vi "WriteUCharImageAttribute.vi"(2 "value":u8[][](array[numeric]), 3 "attribute name":string, 4 "device name":string) -> (0 "error stack":string[](array[string]), 1 "success":bool)   [LabVIEW 2014, in "tango.lvlib"]
uses:
  tango.lvlib
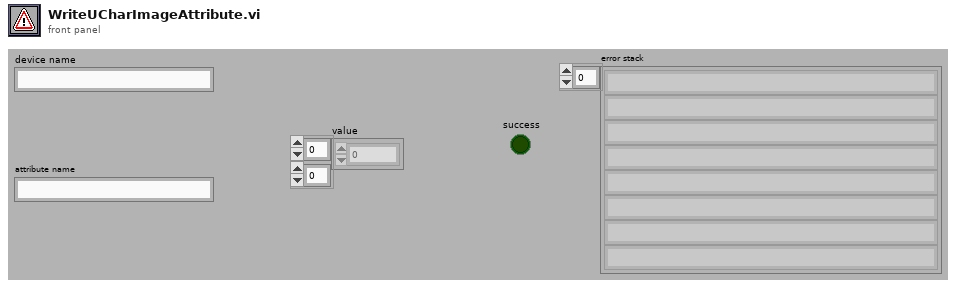
[diagram p1: front panel]
types:
  T1 = cluster{"device name":string, "attribute name":string, "quality value":i16, "quality string":string, "timestamp":dbl, "dim. x":i32, "dim. y":i32, "value":u8[], "error code":i32, "error stack":string[], "data type":u16}
  T2 = cluster{"device name":string, "attribute name":string, "quality value":i16, "quality string":string, "timestamp":dbl, "dim. x":i32, "dim. y":i32, "value":u8[], "error code":i32, "error stack":string[], "data type":u16}[]
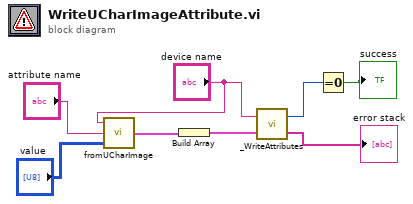
[diagram p0: block diagram]
diagram:
  n1 = call "fromUCharImage.vi"("value"="value", "attribute name"="attribute name", "device name"="device name") -> ("attribute value"=w2:T1)
  n2 = Build Array(w2) -> (w1:T2)
  n3 = call "_WriteAttributes.vi"("attribute Values"=w1, "device name"="device name") -> ("error stack"=→"error stack":string[], "error code"=w8:i32)
  n4 = Equal To 0?(x=w8) -> (x = 0?=→"success":bool)
